vi "GetDSCValues (deprecated).vi"() -> (3 "cluster":T2)   [LabVIEW 2016]
panel:
  out "cluster 2":T1
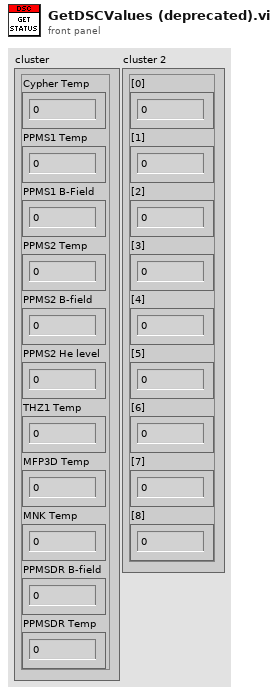
[diagram p1: front panel]
types:
  T1 = cluster{"[0]":dbl, "[1]":dbl, "[2]":dbl, "[3]":dbl, "[4]":dbl, "[5]":dbl, "[6]":dbl, "[7]":dbl, "[8]":dbl}
  T2 = cluster{"Cypher Temp":dbl, "PPMS1 Temp":dbl, "PPMS1 B-Field":dbl, "PPMS2 Temp":dbl, "PPMS2 B-field":dbl, "PPMS2 He level":dbl, "THZ1 Temp":dbl, "MFP3D Temp":dbl, "MNK Temp":dbl, "PPMSDR B-field":dbl, "PPMSDR Temp":dbl}
  T3 = cluster{"PPMS Temp":i32, "PPMS B Field":i32, i32, "Vars":refnum<k21>[]}
  T4 = cluster{"shared variable refnum in":refnum<k21>, "shared variable refnum in 2":refnum<k21>, "shared variable refnum in 3":refnum<k21>, "shared variable refnum in 4":refnum<k21>, "shared variable refnum in 5":refnum<k21>, "shared variable refnum in 6":refnum<k21>, "shared variable refnum in 9":refnum<k21>, "shared variable refnum in 10":refnum<k21>, "shared variable refnum in 11":refnum<k21>, "shared variable refnum in 12":refnum<k21>, "shared variable refnum in 13":refnum<k21>}
  T5 = cluster{"shared variable refnum in 3":refnum<k21>, "shared variable refnum in 4":refnum<k21>, "shared variable refnum in 5":refnum<k21>, "shared variable refnum in 6":refnum<k21>, "shared variable refnum in 9":refnum<k21>, "shared variable refnum in 10":refnum<k21>, "shared variable refnum in 11":refnum<k21>, "shared variable refnum in 12":refnum<k21>, "shared variable refnum in 13":refnum<k21>}
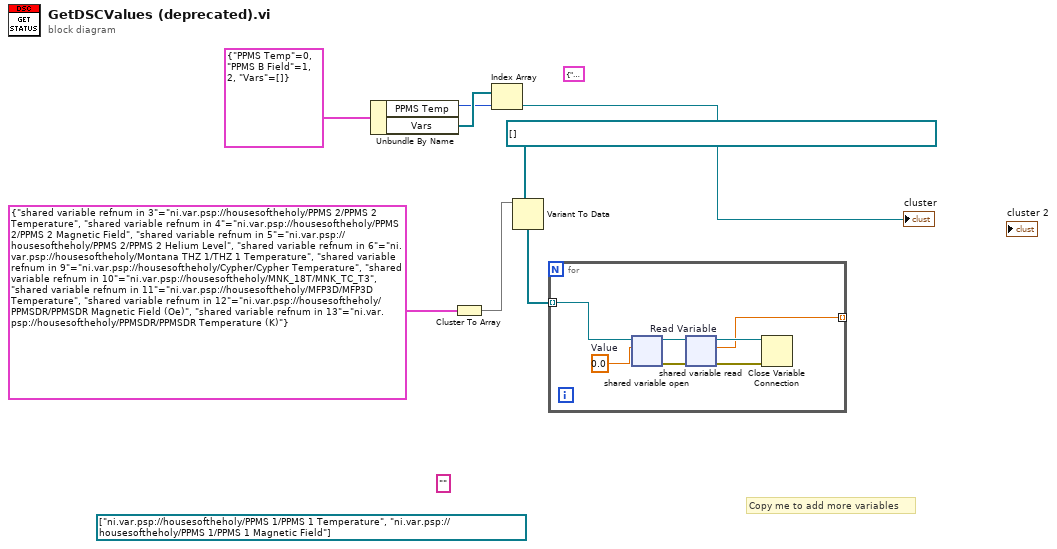
[diagram p0: block diagram]
diagram:
  (unwired) ""
  (unwired) refnum<k21>[] ["ni.var.psp://housesoftheholy/PPMS 1/PPMS 1 Temperature", "ni.var.psp://housesoftheholy/PPMS 1/PPMS 1 Magnetic Field"]
  (unwired) T4 {"shared variable refnum in"="ni.var.psp://housesoftheholy/PPMS 1/PPMS 1 Temperature", "shared variable refnum in 2"="ni.var.psp://housesoftheholy/PPMS 1/PPMS 1 Magnetic Field", "shared variable refnum in 3"="ni.var.psp://housesoftheholy/PPMS 2/PPMS 2 Temperature", "shared variable refnum in 4"="ni.var.psp://housesoftheholy/PPMS 2/PPMS 2 Magnetic Field", "shared variable refnum in 5"="ni.var.psp://housesoftheholy/PPMS 2/PPMS 2 Helium Level", "shared variable refnum in 6"="ni.var.psp://housesoftheholy/Montana THZ 1/THZ 1 Temperature", "shared variable refnum in 9"="ni.var.psp://housesoftheholy/Cypher/Cypher Temperature", "shared variable refnum in 10"="ni.var.psp://housesoftheholy/MNK_18T/MNK_TC_T3", "shared variable refnum in 11"="ni.var.psp://housesoftheholy/MFP3D/MFP3D Temperature", "shared variable refnum in 12"="ni.var.psp://housesoftheholy/PPMSDR/PPMSDR Magnetic Field (Oe)", "shared variable refnum in 13"="ni.var.psp://housesoftheholy/PPMSDR/PPMSDR Temperature (K)"}
  # "Copy me to add more variables"
  n1 = Unbundle By Name(T3 {"PPMS Temp"=0, "PPMS B Field"=1, 2, "Vars"=[]}) -> ("PPMS Temp"=w2:i32, "Vars"=w3:refnum<k21>[])
  n2 = Cluster To Array(cluster=T5 {"shared variable refnum in 3"="ni.var.psp://housesoftheholy/PPMS 2/PPMS 2 Temperature", "shared variable refnum in 4"="ni.var.psp://housesoftheholy/PPMS 2/PPMS 2 Magnetic Field", "shared variable refnum in 5"="ni.var.psp://housesoftheholy/PPMS 2/PPMS 2 Helium Level", "shared variable refnum in 6"="ni.var.psp://housesoftheholy/Montana THZ 1/THZ 1 Temperature", "shared variable refnum in 9"="ni.var.psp://housesoftheholy/Cypher/Cypher Temperature", "shared variable refnum in 10"="ni.var.psp://housesoftheholy/MNK_18T/MNK_TC_T3", "shared variable refnum in 11"="ni.var.psp://housesoftheholy/MFP3D/MFP3D Temperature", "shared variable refnum in 12"="ni.var.psp://housesoftheholy/PPMSDR/PPMSDR Magnetic Field (Oe)", "shared variable refnum in 13"="ni.var.psp://housesoftheholy/PPMSDR/PPMSDR Temperature (K)"}) -> (array=w7:refnum<k21>[])
  n3 = Index Array(array=w3, index=w2) -> (element=→"cluster":refnum<k21>)
  n4 = Variant To Data(type=refnum<k21>[] [], Variant=w7) -> (data=w5:refnum<k21>[])  [unwired: 1 in, 1 out]
  n5 = for {
    tunnel: [w10] -> _ mode=indexing
    tunnel: w5 -> [w9] mode=indexing
    w12 = 0.0  # Value
    n6 = shared-variable-open(w9, w12) -> (w15:refnum<k21>, w13:errorcluster)  [unwired: 2 in]
    n7 = shared-variable-read "Read Variable"(w15, w13) -> (w14:refnum<k21>, w11:errorcluster, w10:dbl)  [unwired: 1 out]
    n8 = Close Variable Connection(8:w11, 11:w14) -> ()  [unwired: 1 out]
  }
